vi "create_directory_structure.vi"(0 "time stamp":timestamp, 1 "File identifier":string) -> (2 "todays path":path, 3 "Basepath":path, 4 "filepath":string)   [LabVIEW 2015]
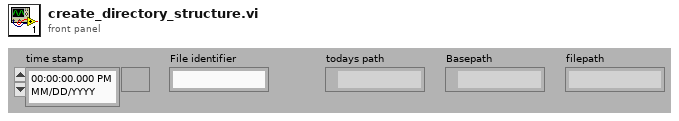
[diagram p1: front panel]
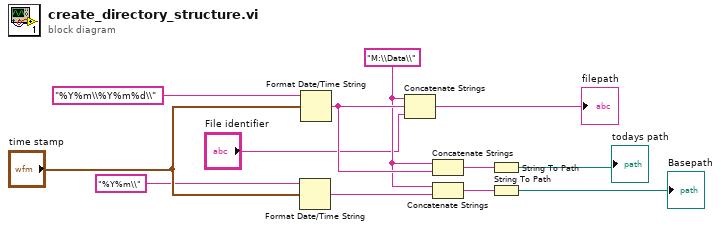
[diagram p0: block diagram]
diagram:
  w2 = "M:\\Data\\" ("string")
  n1 = Format Date/Time String(time format string (%c)="%Y%m\\", seconds (now)="time stamp") -> (date/time string=w7:string)  [unwired: 1 in]
  n2 = Format Date/Time String(time format string (%c)="%Y%m\\%Y%m%d\\", seconds (now)="time stamp") -> (date/time string=w6:string)  [unwired: 1 in]
  n3 = Concatenate Strings(w2, w6, "File identifier") -> (→"filepath":string)
  n4 = Concatenate Strings(w2, w6) -> (w8:string)
  n5 = Concatenate Strings(w2, w7) -> (w5:string)
  n6 = String To Path(string=w8) -> (path=→"todays path":path)
  n7 = String To Path(string=w5) -> (path=→"Basepath":path)
